vi "E1_Conversion_CaF.vi"(1 "Grados C":dbl) -> (0 "Grados F":dbl)   [LabVIEW 2020]
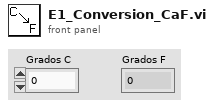
[diagram p1: front panel]
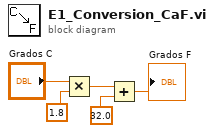
[diagram p0: block diagram]
diagram:
  n1 = Multiply(x="Grados C", y=1.8) -> (x*y=w3:dbl)
  n2 = Add(x=w3, y=32.0) -> (x+y=→"Grados F":dbl)
